vi "Vaporizador_CL.vi"() -> ()   [LabVIEW 2021]
panel:
  in  "Masa":u64
  in  "Sustancia":dbl(ring)=2261.11 items=["Agua", "Alcohol Etílico", "Benceno"]
  out "Gauge":dbl(knob) scale=-10000.0..10000.0
  in  "Detener":bool
  # "VAPORIZADOR"
  # "Calor Necesario"
  # "CONDICIONES"
  # "gr"
  # "kJ"
  # "Desarrollado por:\n     Cesar Augusto Quiñones Segura\n     Andrea Carolina Sanchez Diaz\n     Jhon Erik Navarrete Gómez"
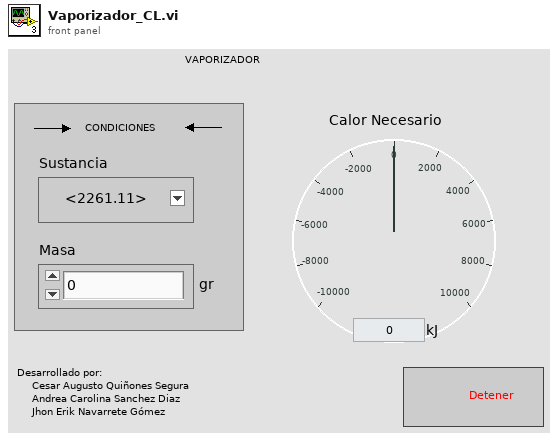
[diagram p1: front panel]
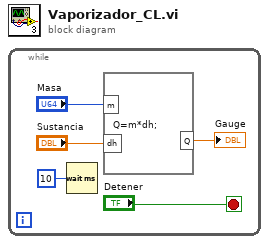
[diagram p0: block diagram]
diagram:
  n1 = while {
    stop <- "Detener" stop-if-true
    n2 = Wait (ms)(milliseconds to wait=u32 10) -> ()  [unwired: 1 out]
    n3 = formula code="Q=m*dh;"("dh"="Sustancia", "m"="Masa") -> ("Q"=→"Gauge":dbl)
  }
